vi "ErrorCatcher.vi"(8 "error in (no error)":errorcluster, 10 "?":T1={"commandlist"="", "line"=0, "last response"="", "timeout"=0, "wait"=0, "erfolgreich"=FALSE, "next state"=enum."Start"}, 11 "CEG4500 in":refnum<class "CEG4500.lvclass">) -> (0 "error out":errorcluster, 3 "CEG4500 out":refnum<class "CEG4500.lvclass">)   [LabVIEW 2013, in "CEG4500.lvclass"]
uses:
  CEG4500.lvclass
  Main/controls/TestData.ctl
  Main/controls/TestStates.ctl
  lib/EMV-Test.lvlib
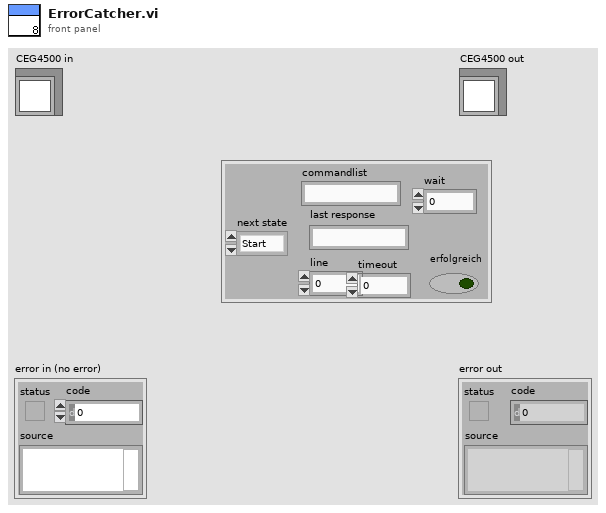
[diagram p1: front panel]
types:
  T1 = typedef "EMV-Test.lvlib/TestData.ctl" = cluster{"commandlist":string, "line":i32, "last response":string, "timeout":i32, "wait":u32, "erfolgreich":bool, "next state":T2}
  T2 = typedef "EMV-Test.lvlib/TestStates.ctl" = enum16{"check for pressed Buttons", "pause", "vorgefertigter Test", "manueller Test", "respond to response", "error", "Start", "Initialise", "open connection", "evaluate line", "wait for Response", "wait", "catch error", "close Connection", "end", "empty buffer"}
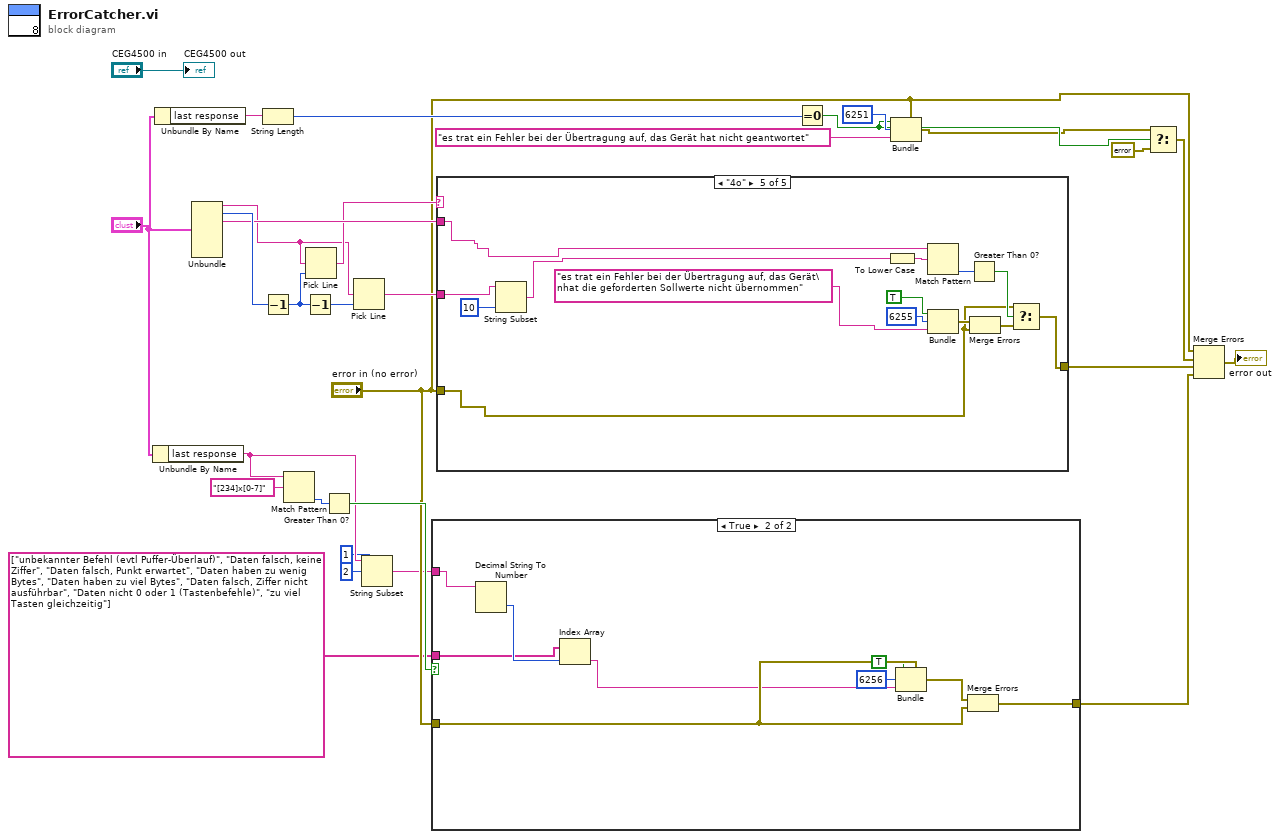
[diagram p0: block diagram]
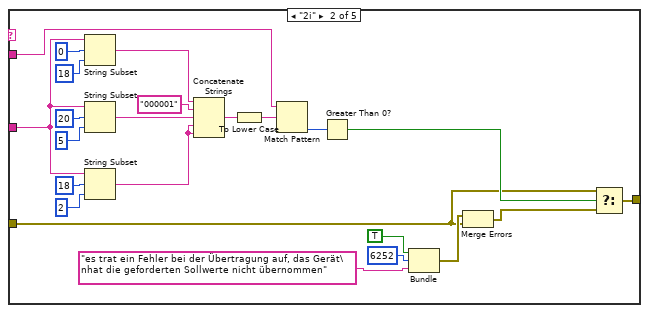
[diagram p4: hidden frame]
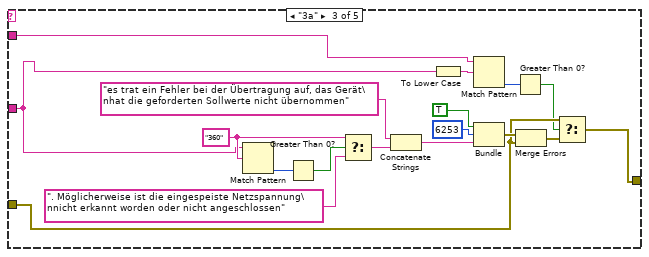
[diagram p5: hidden frame]
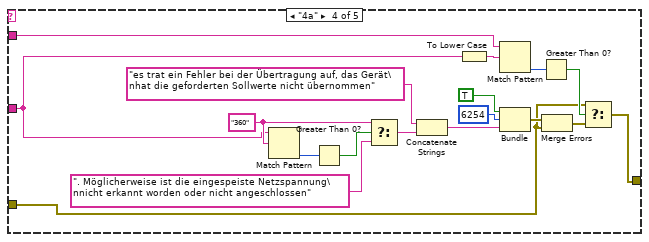
[diagram p6: hidden frame]
diagram:
  n1 = Unbundle By Name("?") -> ("last response"=w6:string)
  n2 = Unbundle By Name("?") -> ("last response"=w21:string)
  n3 = Unbundle("?") -> ("commandlist"=w15:string, "line"=w22:i32, "last response"=w19:string)  [unwired: 4 out]
  n4 = String Length(string=w21) -> (length=w29:i32)
  n5 = Decrement(x=w22) -> (x-1=w17:i32)
  n6 = Match Pattern(string=w6, regular expression="[234]x[0-7]" ("Regulärer Ausdruck")) -> (offset past match=w9:i32)  [unwired: 1 in, 3 out]
  n7 = Decrement(x=w17) -> (x-1=w16:i32)
  n8 = Pick Line(multi-line string=w15, line index=w17) -> (output string=w18:string)  [unwired: 1 in]
  n9 = Greater Than 0?(x=w9) -> (x > 0?=w8:bool)
  n10 = Pick Line(multi-line string=w15, line index=w16) -> (output string=w14:string)  [unwired: 1 in]
  n11 = String Subset(string=w6, offset (0)=2 ("Offset (0)"), length (rest)=1 ("Länge (Rest)")) -> (substring=w3:string)
  n12 = case shown="True" w8 {
    tunnel: "error in (no error)" -> [w30 w36]
    tunnel: w3 -> [_ w39]
    tunnel: string[] ["unbekannter Befehl (evtl Puffer-Überlauf)", "Daten falsch, keine Ziffer", "Daten falsch, Punkt erwartet", "Daten haben zu wenig Bytes", "Daten haben zu viel Bytes", "Daten falsch, Ziffer nicht ausführbar", "Daten nicht 0 oder 1 (Tastenbefehle)", "zu viel Tasten gleichzeitig"] -> [_ w37]
    tunnel: [w30 w31] -> w1
    frame False {
    }
    frame True {
      n13 = Decimal String To Number(string=w39) -> (number=w38:i32)  [unwired: 2 in, 1 out]
      n14 = Index Array(array=w37, index=w38) -> (element=w34:string)
      n15 = Bundle(cluster=w36, "status"=TRUE, "code"=6256, "source"=w34) -> (w35:errorcluster)
      n16 = Merge Errors(w35, w36) -> (w31:errorcluster)
    }
  }
  n17 = case shown="\"4o\"" w18 {
    tunnel: w19 -> [_ w53 w65 w82 w103]
    tunnel: w14 -> [_ w49 w64 w83 w102]
    tunnel: "error in (no error)" -> [w40 w42 w75 w85 w105]
    tunnel: [w40 w41 w74 w84 w106] -> w12
    frame "False", Default {
    }
    frame "2i" {
      n18 = String Subset(string=w49, offset (0)=0, length (rest)=18 ("length (rest)")) -> (substring=w61:string)
      n19 = String Subset(string=w49, offset (0)=20, length (rest)=5 ("length (rest)")) -> (substring=w57:string)
      n20 = String Subset(string=w49, offset (0)=18, length (rest)=2 ("length (rest)")) -> (substring=w54:string)
      n21 = Concatenate Strings(w61, "000001" ("string"), w57, w54, w54) -> (w51:string)
      n22 = To Lower Case(string=w51) -> (all lower case string=w50:string)
      n23 = Match Pattern(string=w53, regular expression=w50) -> (offset past match=w52:i32)  [unwired: 1 in, 3 out]
      n24 = Greater Than 0?(x=w52) -> (x > 0?=w44:bool)
      n25 = Bundle("status"=TRUE, "code"=6252, "source"="es trat ein Fehler bei der Übertragung auf, das Gerät\nhat die geforderten Sollwerte nicht übernommen") -> (w45:errorcluster)  [unwired: 1 in]
      n26 = Merge Errors(w45, w42) -> (w43:errorcluster)
      n27 = Select(t=w42, s=w44, f=w43) -> (s? t:f=w41:errorcluster)
    }
    frame "3a" {
      w68 = "360" ("regular expression")
      n28 = Match Pattern(string=w64, regular expression=w68) -> (offset past match=w72:i32)  [unwired: 1 in, 3 out]
      n29 = Greater Than 0?(x=w72) -> (x > 0?=w69:bool)
      n30 = Select(t=w68, s=w69, f=". Möglicherweise ist die eingespeiste Netzspannung\nnicht erkannt worden oder nicht angeschlossen") -> (s? t:f=w66:string)
      n31 = Concatenate Strings("es trat ein Fehler bei der Übertragung auf, das Gerät\nhat die geforderten Sollwerte nicht übernommen" ("source"), w66) -> (w70:string)
      n32 = To Lower Case(string=w64) -> (all lower case string=w81:string)
      n33 = Match Pattern(string=w65, regular expression=w81) -> (offset past match=w80:i32)  [unwired: 1 in, 3 out]
      n34 = Bundle("status"=TRUE, "code"=6253, w70) -> (w77:cluster{"status":bool, "code":i32, string})  [unwired: 1 in]
      n35 = Greater Than 0?(x=w80) -> (x > 0?=w73:bool)
      n36 = Merge Errors(w77, w75) -> (w76:errorcluster)
      n37 = Select(t=w75, s=w73, f=w76) -> (s? t:f=w74:errorcluster)
    }
    frame "4a" {
      w88 = "360" ("regular expression")
      n38 = Match Pattern(string=w83, regular expression=w88) -> (offset past match=w92:i32)  [unwired: 1 in, 3 out]
      n39 = Greater Than 0?(x=w92) -> (x > 0?=w89:bool)
      n40 = Select(t=w88, s=w89, f=". Möglicherweise ist die eingespeiste Netzspannung\nnicht erkannt worden oder nicht angeschlossen") -> (s? t:f=w86:string)
      n41 = Concatenate Strings("es trat ein Fehler bei der Übertragung auf, das Gerät\nhat die geforderten Sollwerte nicht übernommen" ("source"), w86) -> (w90:string)
      n42 = To Lower Case(string=w83) -> (all lower case string=w99:string)
      n43 = Match Pattern(string=w82, regular expression=w99) -> (offset past match=w98:i32)  [unwired: 1 in, 3 out]
      n44 = Bundle("status"=TRUE, "code"=6254, w90) -> (w95:cluster{"status":bool, "code":i32, string})  [unwired: 1 in]
      n45 = Greater Than 0?(x=w98) -> (x > 0?=w93:bool)
      n46 = Merge Errors(w95, w85) -> (w94:errorcluster)
      n47 = Select(t=w85, s=w93, f=w94) -> (s? t:f=w84:errorcluster)
    }
    frame "4o" {
      n48 = String Subset(string=w102, length (rest)=10 ("length (rest)")) -> (substring=w100:string)  [unwired: 1 in]
      n49 = To Lower Case(string=w100) -> (all lower case string=w113:string)
      n50 = Match Pattern(string=w103, regular expression=w113) -> (offset past match=w112:i32)  [unwired: 1 in, 3 out]
      n51 = Bundle("status"=TRUE, "code"=6255, "source"="es trat ein Fehler bei der Übertragung auf, das Gerät\nhat die geforderten Sollwerte nicht übernommen") -> (w109:errorcluster)  [unwired: 1 in]
      n52 = Greater Than 0?(x=w112) -> (x > 0?=w107:bool)
      n53 = Merge Errors(w109, w105) -> (w108:errorcluster)
      n54 = Select(t=w105, s=w107, f=w108) -> (s? t:f=w106:errorcluster)
    }
  }
  n55 = Equal To 0?(x=w29) -> (x = 0?=w26:bool)
  n56 = Bundle(cluster="error in (no error)", "status"=w26, "code"=6251, "source"="es trat ein Fehler bei der Übertragung auf, das Gerät hat nicht geantwortet") -> (w25:errorcluster)
  n57 = Select(t=w25, s=w26, f=errorcluster {"status"=FALSE, "code"=0, "source"=""}) -> (s? t:f=w23:errorcluster)
  n58 = Merge Errors("error in (no error)", w23, w12, w1) -> (→"error out":errorcluster)
  "CEG4500 out" <- "CEG4500 in"
